vi "SOS_Global_2022.vi"() -> ()   [LabVIEW 2016]
panel:
  in  "C source ref water":i32(listbox)
  in  "C source ref dry air":i32(listbox)=1
  in  "Bdw source air-water interaction virial":i32(listbox)=3
  in  "Bw source ref water":i32(listbox)=2
  in  "Bd source ref dry air":i32(listbox)=1
  in  "CO2 content / ppm":dbl=500.0
  in  "Type of air":i32(listbox)=4
  in  "Frequency":dbl=10.0
  in  "Humidity":dbl=50.0 format="%.3f"
  in  "Pressure":dbl=1.0 format="%.3f"
  in  "frequency unit":i32(listbox)=1
  in  "humidity unit":i32(listbox)=3
  in  "Pressure unit":i32(listbox)=2
  in  "Temperature unit":i32(listbox)
  in  "Temperature":dbl=373.15 format="%.4g"
  in  "gamma s":dbl=1.364192475474738 format="%#_8g"
  in  "SoS Kr [m/s]":dbl
  in  "SoS Kv [m/s]":dbl
  in  "SoS Kc [m/s]":dbl
  in  "Simple SoS [m/s]":dbl
  in  "K_v vir corr":dbl=-0.0047447288095566025
  in  "K_c c spec corr":dbl=-0.005905811453997711
  in  "3 Ac press Vir Mix [G]":dbl=-1.6549788810026356e-14
  in  "gamma0wa":dbl=1.356135811927622
  in  "gamma0wT":dbl=1.323128876046848 format="%#.17g"
  in  "gamma0aT":dbl=1.3968263453872474 format="%#_8g"
  in  "Cw(T)":dbl=-4.4682461395292936e-07
  in  "Ca(T)":dbl=1.219835549278853e-09
  in  "Cmix(xw,T) [m^3/mol]^2":dbl=-5.6022981207138925e-08
  in  "d^2Cw/dT^2":dbl
  in  "d^2Ca/dT^2":dbl=2.3734887970956986e-15
  in  "dCw/dT":dbl=-7.456356433944506e-14
  in  "dCa/dT":dbl=-9.989510208451924e-13
  in  "Lch":dbl=-1.2307824264948054e-06
  in  "Lcd":dbl=3.077772643787857e-09
  in  "Lbbh":dbl=-0.000850382289081476
  in  "Lbbd":dbl=4.162623275226506e-05
  in  "2 Ac press Vir Mix [F]":dbl=-4.514992521291588e-08
  in  "K mix":dbl=-0.00014007952659137997
  in  "Kw":dbl=-0.0005889340832523563
  in  "Ka":dbl=3.0070758323398767e-05
  in  "d^2Bw(T)/dT^2":dbl=-7.054453286930115e-08
  in  "d^2Ba(T)/dT^2":dbl=-7.083723741101137e-10
  in  "dBw(T)/dT":dbl=4.517709644341583e-06
  in  "dBa(T)/dT":dbl=1.1544291063273333e-07
  in  "Bmix(T)":dbl=-0.00011942556999113059
  in  "Bw(T)":dbl=-0.00045162277028342796
  in  "Ba(T)":dbl=3.5008568678367798e-06
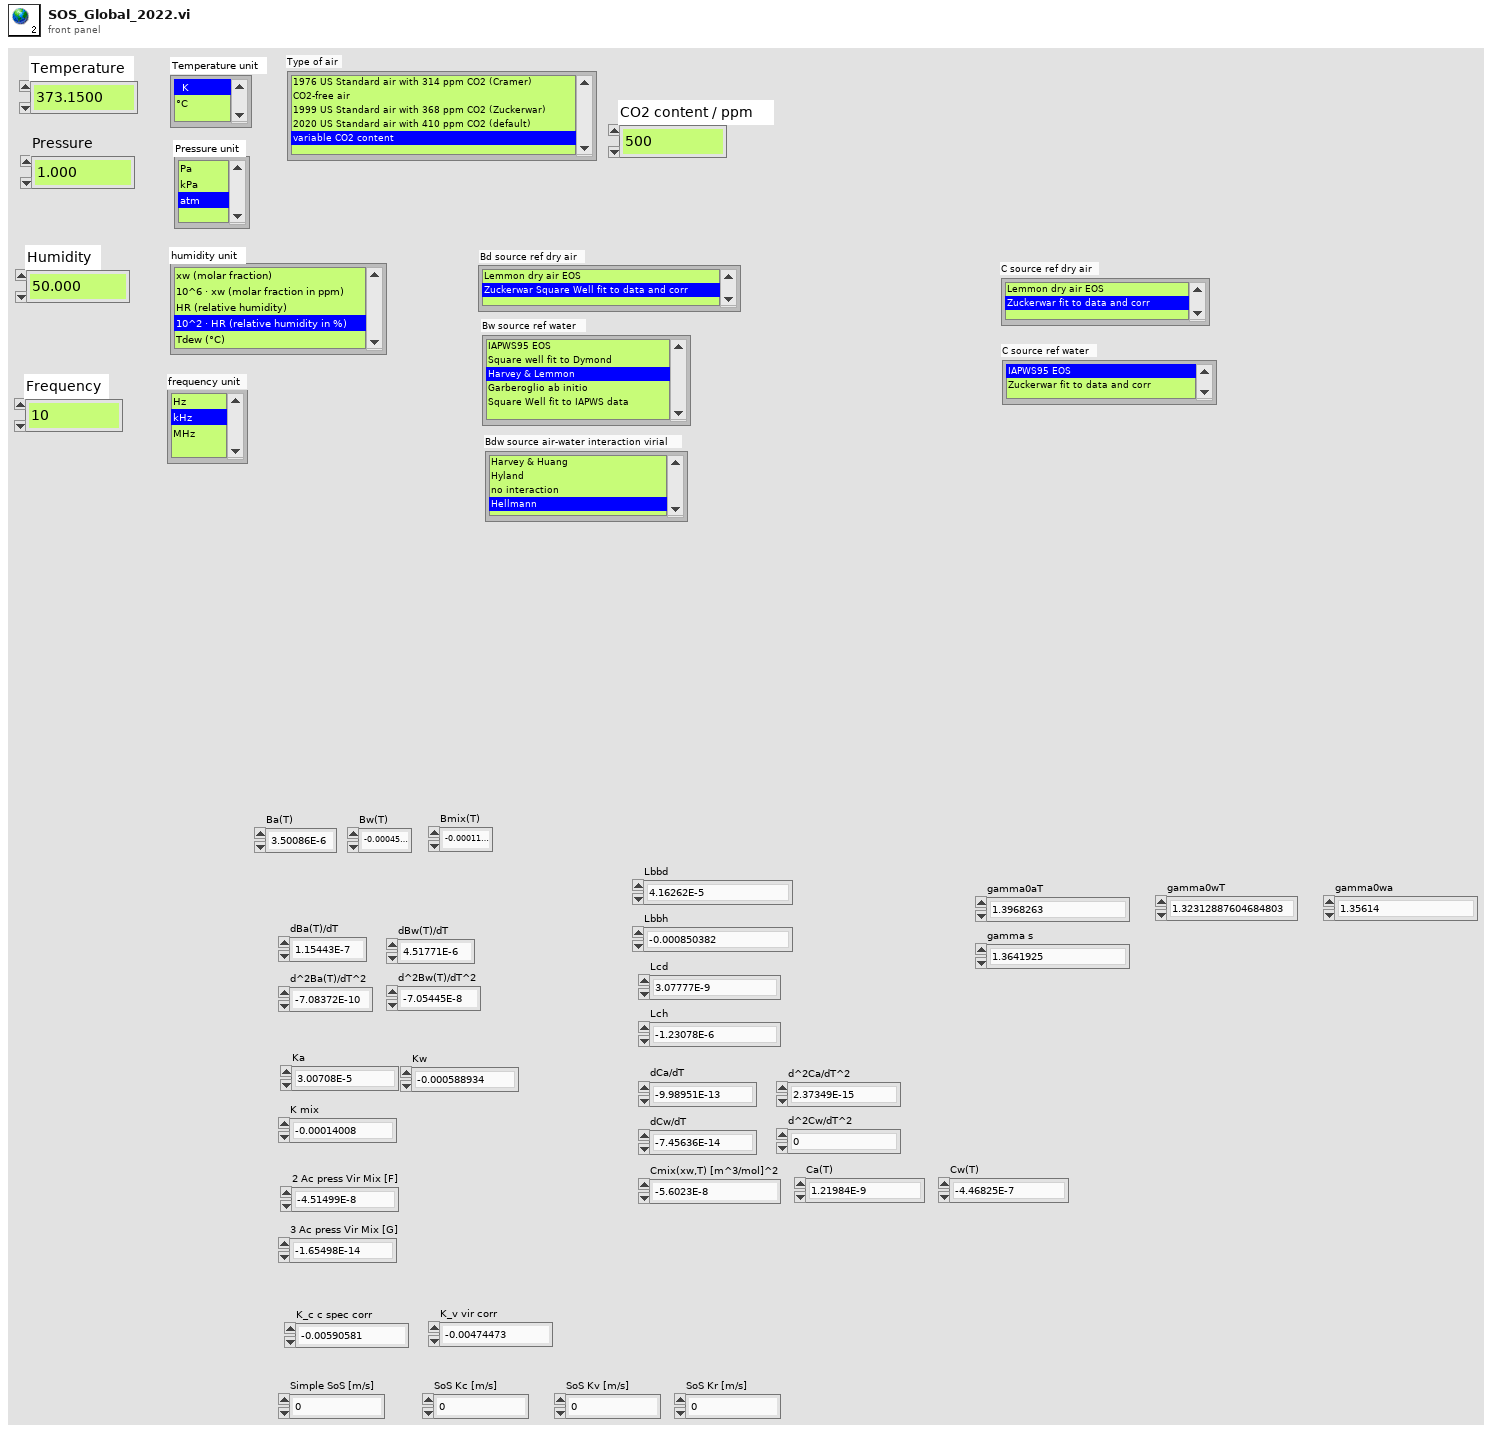
[diagram p1: front panel]
diagram:
